vi "configuration UI.vi"() -> ()   [LabVIEW 2013, in "Tag Bus Web Interface editor node.lvclass"]
uses:
  Tag Bus Web Interface editor node.lvclass
  <vilib>/CEF_TreeControl/Node/NodeRef.ctl
  <vilib>/CEF_TreeControl/Node/NISE_CEF_Node.lvclass
  <vilib>/NI/AMC/Message Queue.ctl
  <vilib>/NI/AMC/Message.ctl
  <vilib>/NI/Tools/Keyed Array/KeyedArray.ctl
  <vilib>/CEF_TreeControl/Node/UserEventRef.ctl
  <vilib>/CEF_TreeControl/Controls/EventCluster.ctl
  <vilib>/NI/Module Execution Interface/Engine Configuration/engine configuration.lvclass
  <vilib>/NI/Tag Bus Data Framework/Configuration Editor/Classes/Engine Parent/Engine Parent Editor Node.lvclass
  <vilib>/NI/TBM Modules/TBWI/configuration/Tag Bus Web Interface configuration.lvclass
  <vilib>/NI/Tag Bus/tag/tag descriptor.lvclass
  <vilib>/NI/Tag Bus/tag/Data Type.ctl
  <vilib>/NI/Tag Bus/tag/tag descriptor.lvclass/tag descriptor.ctl
  Tag Bus Web Interface editor node.lvclass/Tag Bus Web Interface editor node.ctl
  <vilib>/NI/Tag Bus Module Framework/root configuration/TBM configuration.lvclass/TBM configuration.ctl
  <vilib>/NI/Tag Bus Module Framework/channel/channel classification.ctl
  <vilib>/NI/Tag Bus/tag/write tag name.vi
  <vilib>/NI/Tag Bus/tag/write data type.vi
  <vilib>/NI/Tag Bus/tag/read tag name.vi
  <vilib>/NI/Tag Bus Data Framework/Configuration Editor/Classes/Engine Parent/read engine configuration.vi
  <vilib>/NI/Tag Bus Module Framework/root configuration/create GUID.vi
  <vilib>/NI/Tag Bus Data Framework/Configuration Editor/Classes/Engine Parent/write engine configuration.vi
  <vilib>/NI/Tag Bus Module Framework/root configuration/TBM configuration.lvclass
  <vilib>/NI/Tag Bus Data Framework/Configuration Editor/Classes/Module editor node/module editor node.lvclass
  <vilib>/CEF_TreeControl/NISE_CEF_TreeControl.lvlib
  <vilib>/NI/Tag Bus Module Framework/channel/TBM channel.lvclass
  <vilib>/NI/Tools/Keyed Array/Tools_KeyedArray.lvlib
  <vilib>/NI/AMC/AMC.lvlib
panel:
  in  "Tab Control":enum32{"Web Configuration"}(tab)
  in  "remove to":bool
  in  "add to":bool
  in  "remove from":bool
  in  "add from":bool
  in  "toTBWlist":i32(listbox)
  in  "fromTBWlist":i32(listbox)
  in  "avail tags":i32(listbox)=-1
  in  "Direction":enum32{"From TBWI", "To TBWI"}(radio)
  in  "user event":T1
  in  "main queue":T2
  in  "node ref":T3
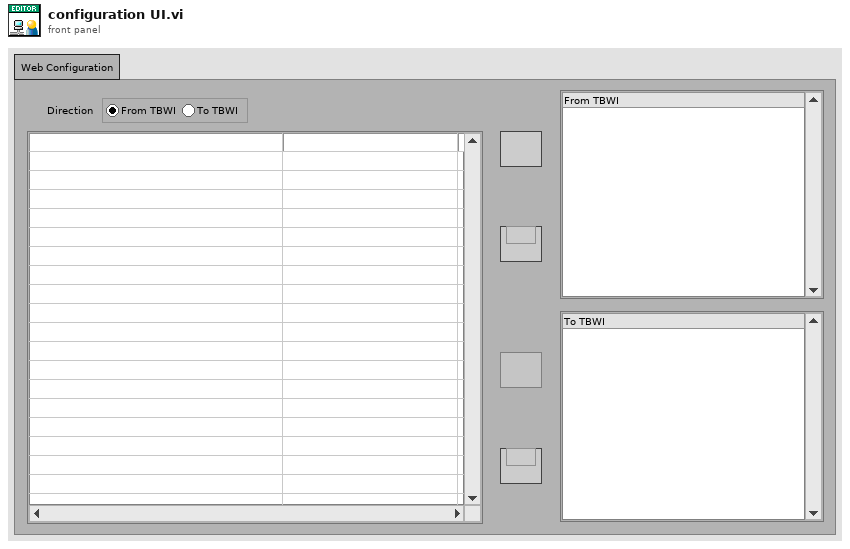
[diagram p1: front panel]
types:
  T1 = typedef "NISE_CEF_Node.lvclass/UserEventRef.ctl" = refnum<user-event>
  T2 = typedef "AMC.lvlib/Message Queue.ctl" = refnum<queue>
  T3 = typedef "NISE_CEF_Node.lvclass/NodeRef.ctl" = refnum<data-value>
  T4 = typedef "NISE_CEF_TreeControl.lvlib/EventCluster.ctl" = cluster{"command":string, "data":string}
  T5 = typedef "tag bus.lvlib/tag descriptor.lvclass/Data Type.ctl" = enum16{"Double", "Single", "I64", "I32", "I16", "I8", "U64", "U32", "U16", "U8", "Boolean", "String", "Array of Double", "Array of Single", "Array of I64", "Array of I32", "Array of I16", "Array of I8", "Array of U64", "Array of U32", "Array of U16", "Array of U8", "Array of Boolean", "Array of String"}
  T6 = enum8{"Enabled", "Disabled", "Disabled and Grayed Out"}
  T7 = typedef "TBM channel.lvclass/channel classification.ctl" = enum16{"input data", "output data", "processing parameter", "processing result"}
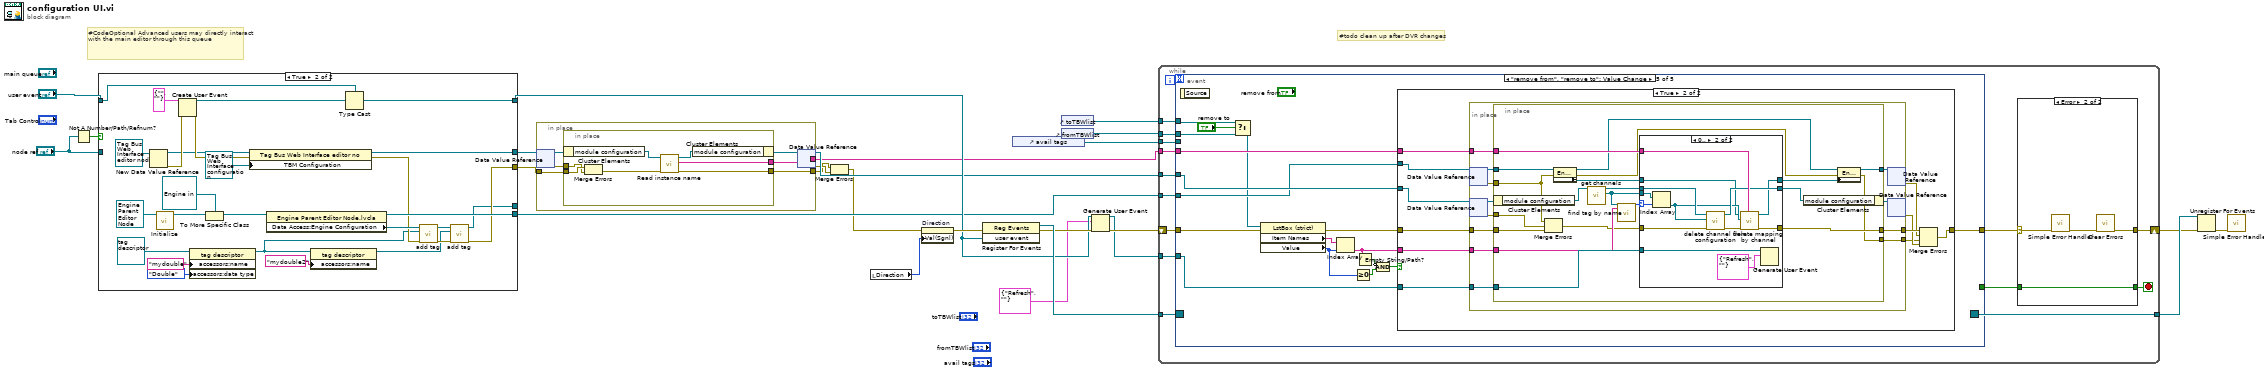
[diagram p0: block diagram]
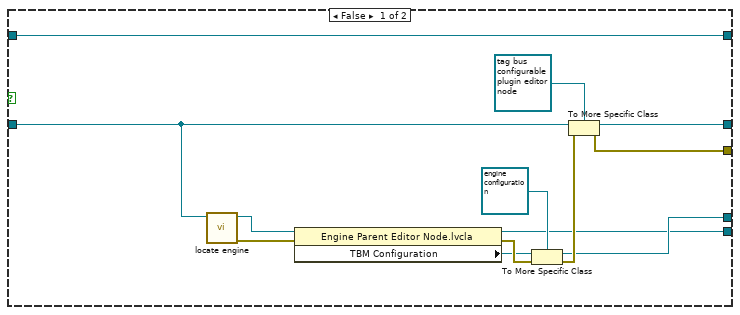
[diagram p2: hidden frame]
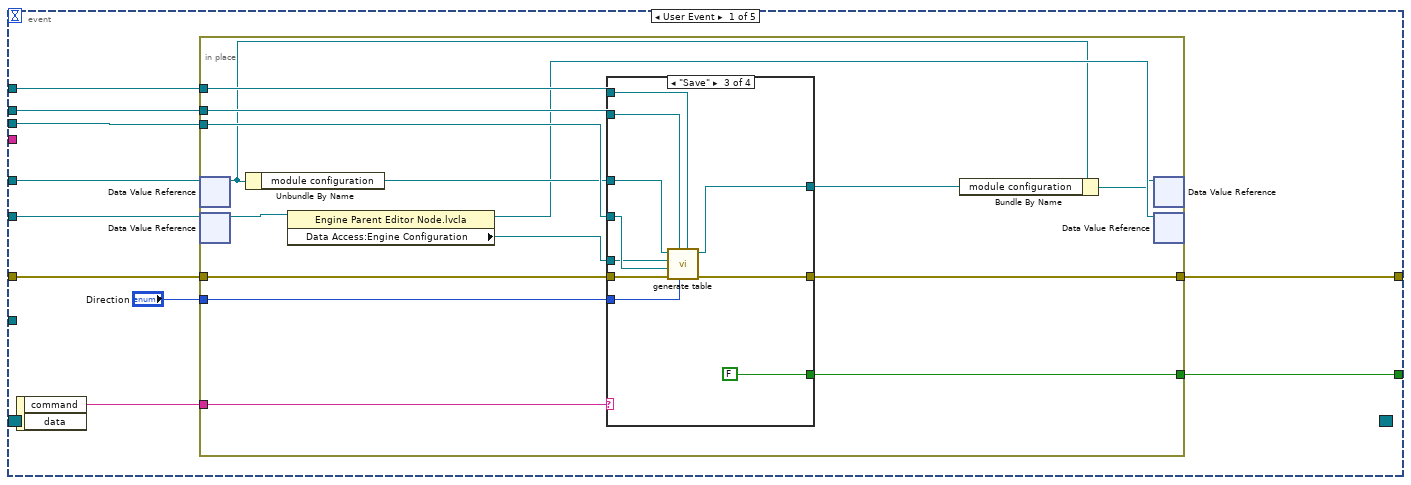
[diagram p4: hidden frame]
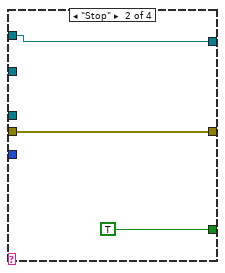
[diagram p6: hidden frame]
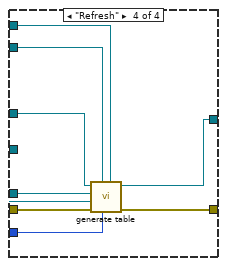
[diagram p7: hidden frame]
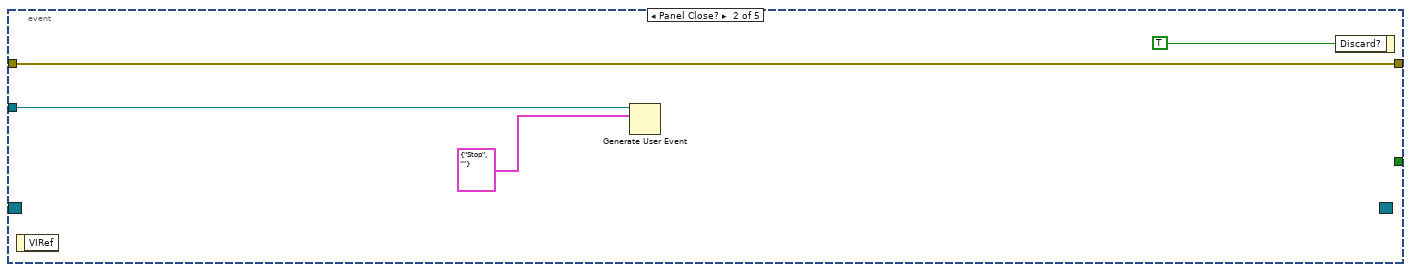
[diagram p8: hidden frame]
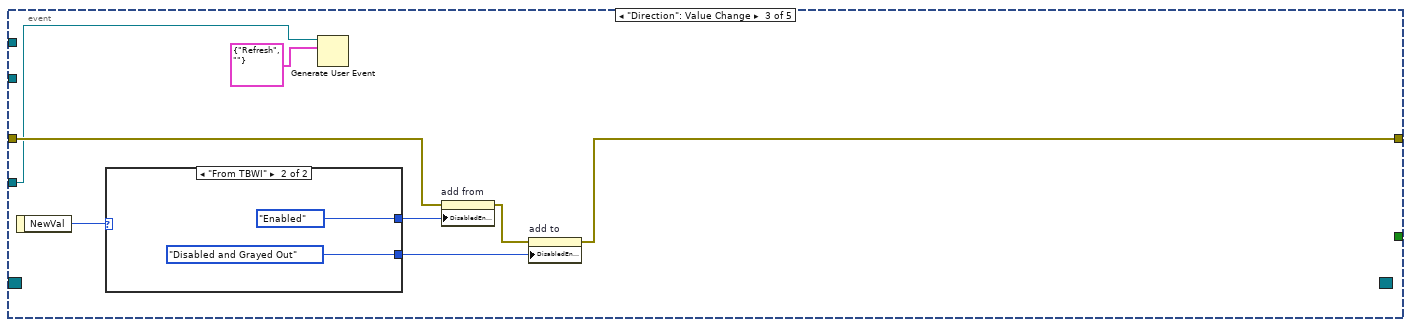
[diagram p9: hidden frame]
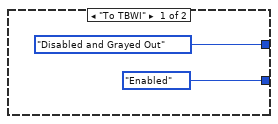
[diagram p10: hidden frame]
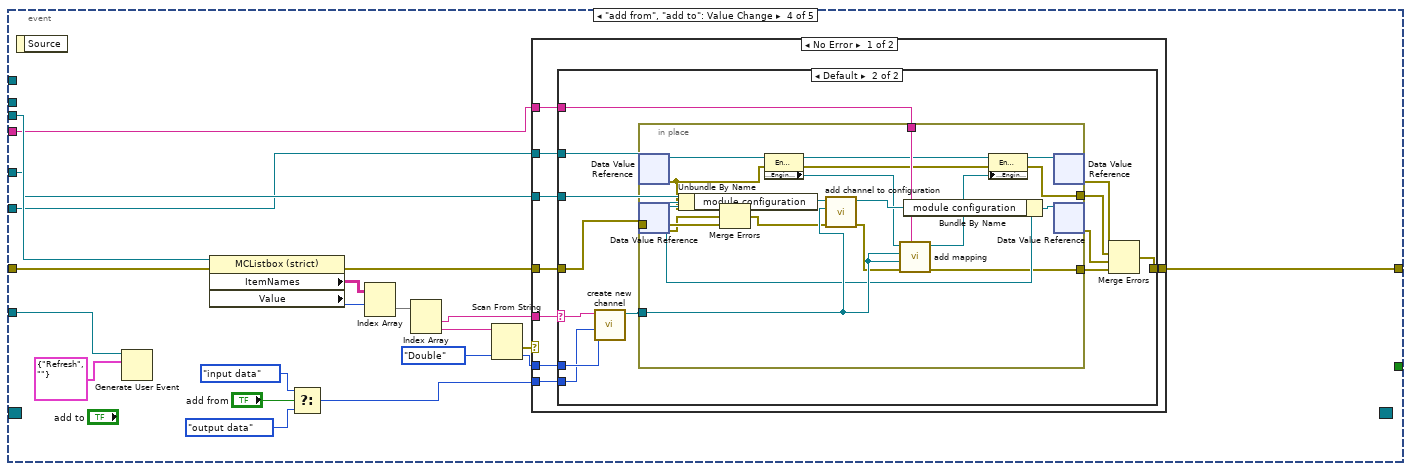
[diagram p11: hidden frame]
diagram:
  # "#todo clean up after DVR changes"
  # "#CodeOptional Advanced users may directly interact with the main editor through this queue"
  n1 = Not A Number/Path/Refnum?(number/path/refnum="node ref") -> (NaN/Path/Refnum?=w22:bool)
  n2 = case shown="True" w22 {
    tunnel: "user event" -> [w38 w39]
    tunnel: [w38 w40] -> w11
    tunnel: "node ref" -> [w36 _]
    tunnel: [w35 w59] -> w7
    tunnel: [w34 w44] -> w5
    tunnel: [w27 w43] -> _
    tunnel: [w26 w53] -> w8
    frame False {
      n3 = call <vilib>:"locate engine.vi"("component"=w36) -> ("error out"=w31:errorcluster, "engine"=w33:refnum<data-value>)  [unwired: 9 in]
      n4 = property class="Engine Parent Editor Node.lvcla"(reference=w33, error in=w31) -> (reference out=w26:refnum<data-value>, error out=w30:errorcluster, "TBM Configuration"=w29:refnum<class "TBM configuration.lvclass">)
      n5 = To More Specific Class(target class=refnum<class "engine configuration.lvclass"> refnum ("engine configuration.lvclass"), reference=w29, error in=w30) -> (specific class reference=w27:refnum<class "engine configuration.lvclass">, error out=w28:errorcluster)
      n6 = To More Specific Class(target class=refnum<data-value> refnum ("data value reference"), reference=w36, error in=w28) -> (specific class reference=w35:refnum<data-value>, error out=w34:errorcluster)
    }
    frame True {
      n7 = New Data Value Reference(data value=refnum<class "Tag Bus Web Interface editor node.lvclass"> refnum ("tag bus configurable plugin editor node")) -> (data value reference=w58:refnum<data-value>, error out=w61:errorcluster)  [unwired: 1 in]
      n8 = call-dynamic "Initialize.vi"("Engine in"=refnum<class "Engine Parent Editor Node.lvclass"> refnum) -> ("data value reference"=w57:T3)  [unwired: 8 in, 2 out]
      n9 = Create User Event(user event datatype=T4 {"command"="", "data"=""} ("event data"), error in=w61) -> (user event=w64:refnum<user-event>, error out=w60:errorcluster)
      n10 = property class="tag descriptor"(reference=refnum<class "tag descriptor.lvclass"> refnum ("tag descriptor"), "accessors:name"="mydouble" ("name"), "accessors:data type"=Data_Type."Double" ("data type")) -> (reference out=w41:refnum<class "tag descriptor.lvclass">)  [unwired: 1 in, 1 out]
      n11 = To More Specific Class(target class=refnum<data-value> refnum ("data value reference"), reference=w57) -> (specific class reference=w56:refnum<data-value>)  [unwired: 1 in, 1 out]
      n12 = property class="Tag Bus Web Interface editor no"(reference=w58, error in=w60, "TBM Configuration"=refnum<class "Tag Bus Web Interface configuration.lvclass"> refnum ("tag bus configurable plugin module configuration")) -> (reference out=w59:refnum<data-value>, error out=w48:errorcluster)
      n13 = property class="Engine Parent Editor Node.lvcla"(reference=w56) -> (reference out=w53:refnum<data-value>, "Data Access:Engine Configuration"=w52:refnum<class "engine configuration.lvclass">)  [unwired: 1 in, 1 out]
      n14 = property class="tag descriptor"(reference=w41, "accessors:name"="mydouble2" ("name")) -> (reference out=w42:refnum<class "tag descriptor.lvclass">)  [unwired: 1 in, 1 out]
      n15 = Type Cast(type=w39, x=w64) -> (*(type *) &x=w40:T1)
      n16 = call <vilib>:"add tag.vi"("error in"=w48, "tag descriptor"=w41, "engine configuration in"=w52) -> ("error out"=w46:errorcluster, "engine configuration out"=w45:refnum<class "engine configuration.lvclass">)  [unwired: 7 in]
      n17 = call <vilib>:"add tag.vi"("error in"=w46, "tag descriptor"=w42, "engine configuration in"=w45) -> ("error out"=w44:errorcluster, "engine configuration out"=w43:refnum<class "engine configuration.lvclass">)  [unwired: 7 in]
    }
  }
  n18 = in-place {
    in-place-border: w5 -> [w69]
    in-place-border: [w68] -> w3
    in-place-border: [w67] -> w2
    n19 = in-place-dvr #1(w7) -> (w71:refnum<class "Tag Bus Web Interface editor node.lvclass">, w70:errorcluster)
    n20 = in-place {
      in-place-border: w70 -> [w77]
      in-place-border: w69 -> [w78]
      in-place-border: [w73] -> w68
      in-place-border: [w72] -> w67
      n21 = in-place-cluster #2(w71) -> ("module configuration"=w76:refnum<class "Tag Bus Web Interface configuration.lvclass">)
      n22 = Merge Errors(w78, w77) -> (w74:errorcluster)
      n23 = call <vilib>:"Read instance name.vi"("error in"=w74, "configuration in"=w76) -> ("error out"=w73:errorcluster, "instance id"=w72:string, "configuration out"=w75:refnum<class "Tag Bus Web Interface configuration.lvclass">)  [unwired: 7 in]
      n24 = in-place-cluster #2("module configuration"=w75) -> (w66:refnum<class "Tag Bus Web Interface editor node.lvclass">)
    }
    n25 = in-place-dvr #1(w66) -> (w6:refnum<data-value>, w4:errorcluster)
  }
  n26 = Merge Errors(w3, w4) -> (w1:errorcluster)
  n27 = local read "Direction"() -> (w13:enum32{"From TBWI", "To TBWI"})
  n28 = property on="Direction" class="RadioBtnsControl (strict)"(error in=w1, "Val(Sgnl)"=w13) -> (error out=w14:errorcluster)  [unwired: 1 in, 1 out]
  n29 = register-events(error in=w14, w11) -> (reference out=w25:refnum<event-registration>, error out=w19:errorcluster)  [unwired: 1 in]
  n30 = control-ref of="avail tags"() -> (w17:refnum<vi>)
  n31 = control-ref of="toTBWlist"() -> (w16:refnum<vi>)
  n32 = control-ref of="fromTBWlist"() -> (w15:refnum<vi>)
  n33 = Generate User Event(user event=w11, event data cluster=T4 {"command"="Refresh", "data"=""} ("event data"), error in=w19) -> (user event out=w10:T1, error out=w12:errorcluster)  [unwired: 1 in]
  n34 = while {
    tunnel: w25 -> [w92]
    tunnel: [w91] -> w24
    shift-right: [w87] -> w23
    shift-left: w12 -> [w90]
    tunnel: w2 -> [w84]
    tunnel: w17 -> [w82]
    tunnel: w10 -> [w81]
    tunnel: w16 -> [w80]
    tunnel: w15 -> [w79]
    tunnel: w6 -> [w86]
    tunnel: w8 -> [w85]
    stop <- w89 stop-if-true
    n35 = event shown="[4] \"remove from\", \"remove to\": Value Change" {
      selector: w92 -> [_ _ _ _ _]
      dyn-events: [_ _ _ _ _] -> w91
      timeout: _ -> [_ _ _ _ _]
      tunnel: [w108 _ _ _ _] -> w88
      tunnel: [w106 w151 w154 w165 w233] -> w83
      tunnel: w90 -> [w105 w151 w155 w170 w228]
      tunnel: w86 -> [w100 _ _ w168 w232]
      tunnel: w85 -> [w99 _ _ w167 w231]
      tunnel: w84 -> [_ _ _ w166 w230]
      tunnel: w82 -> [w104 _ _ w169 _]
      tunnel: w81 -> [_ w149 w152 w184 w227]
      tunnel: w80 -> [w102 _ _ _ w243]
      tunnel: w79 -> [w103 _ _ _ w241]
      event User Event {
        n36 = event-data() -> ("command"=w107:string)  [unwired: 1 in, 1 out]
        n37 = in-place {
          in-place-border: [w123] -> w108
          in-place-border: w107 -> [w122]
          in-place-border: [w121] -> w106
          in-place-border: w105 -> [w120]
          in-place-border: w104 -> [w119]
          in-place-border: w103 -> [w118]
          in-place-border: w102 -> [w117]
          in-place-border: "Direction" -> [w116]
          n38 = in-place-dvr #3(w100) -> (w111:refnum<class "Tag Bus Web Interface editor node.lvclass">)  [unwired: 1 out]
          n39 = in-place-dvr #4(w99) -> (w115:refnum<class "Engine Parent Editor Node.lvclass">)  [unwired: 1 out]
          n40 = Unbundle By Name(w111) -> ("module configuration"=w114:refnum<class "Tag Bus Web Interface configuration.lvclass">)
          n41 = property class="Engine Parent Editor Node.lvcla"(reference=w115) -> (reference out=w112:refnum<class "Engine Parent Editor Node.lvclass">, "Data Access:Engine Configuration"=w113:refnum<class "engine configuration.lvclass">)  [unwired: 1 in, 1 out]
          n42 = case shown="\"Save\"" w122 {
            tunnel: [_ TRUE FALSE _] -> w123
            tunnel: [w125 w127 w132 w146] -> w121
            tunnel: w120 -> [w125 w127 w137 w147]
            tunnel: w119 -> [_ _ w134 w142]
            tunnel: w118 -> [_ _ w135 w145]
            tunnel: w117 -> [_ _ w136 w144]
            tunnel: w116 -> [_ _ w133 w143]
            tunnel: w114 -> [w124 w126 w131 w140]
            tunnel: w113 -> [_ _ w130 w139]
            tunnel: [w124 w126 w129 w141] -> w110
            frame Default {
            }
            frame "Stop" {
            }
            frame "Save" {
              n43 = call "generate table.vi"("to tbwi"=w136, "Direction"=w133, "from tbwi"=w135, "error in"=w137, "tags"=w134, "engine configuration in"=w130, "Tag Bus Web Interface configuration in"=w131) -> ("error out"=w132:errorcluster, "TBWI Cfg out"=w129:refnum<class "Tag Bus Web Interface configuration.lvclass">)  [unwired: 3 in]
            }
            frame "Refresh" {
              n44 = call "generate table.vi"("to tbwi"=w144, "Direction"=w143, "from tbwi"=w145, "error in"=w147, "tags"=w142, "engine configuration in"=w139, "Tag Bus Web Interface configuration in"=w140) -> ("error out"=w146:errorcluster, "TBWI Cfg out"=w141:refnum<class "Tag Bus Web Interface configuration.lvclass">)  [unwired: 3 in]
            }
          }
          n45 = Bundle By Name(cluster=w111, "module configuration"=w110) -> (w109:refnum<class "Tag Bus Web Interface editor node.lvclass">)
          n46 = in-place-dvr #3(w109) -> ()  [unwired: 2 out]
          n47 = in-place-dvr #4(w112) -> ()  [unwired: 2 out]
        }
      }
      event Panel Close? {
        n48 = event-data() -> ()  [unwired: 1 in, 1 out]
        n49 = Generate User Event(user event=w149, event data cluster=T4 {"command"="Stop", "data"=""} ("event data")) -> ()  [unwired: 2 in, 2 out]
        n50 = event-data("Discard?"=TRUE) -> ()  [unwired: 1 in, 1 out]
      }
      event "Direction": Value Change {
        n51 = event-data() -> ("NewVal"=w159:enum32{"From TBWI", "To TBWI"})  [unwired: 1 in]
        n52 = case shown="\"From TBWI\"" w159 {
          tunnel: [T6."Disabled and Grayed Out" ("Disabled") T6."Enabled" ("Disabled")] -> w158
          tunnel: [T6."Enabled" ("Disabled") T6."Disabled and Grayed Out" ("Disabled")] -> w157
          frame "To TBWI" {
          }
          frame "From TBWI" {
          }
        }
        n53 = Generate User Event(user event=w152, event data cluster=T4 {"command"="Refresh", "data"=""} ("event data")) -> ()  [unwired: 2 in, 2 out]
        n54 = property on="add from" class="Bool"(error in=w155, "DisabledEnum"=w158) -> (error out=w156:errorcluster)  [unwired: 1 in, 1 out]
        n55 = property on="add to" class="Bool"(error in=w156, "DisabledEnum"=w157) -> (error out=w154:errorcluster)  [unwired: 1 in, 1 out]
      }
      event "add from", "add to": Value Change {
        n56 = event-data() -> ()  [unwired: 1 in, 1 out]
        n57 = Generate User Event(user event=w184, event data cluster=T4 {"command"="Refresh", "data"=""} ("event data")) -> ()  [unwired: 2 in, 2 out]
        n58 = property class="MCListbox (strict)"(reference=w169, error in=w170) -> (error out=w171:errorcluster, "ItemNames"=w172:string[][], "Value"=w173:i32)  [unwired: 1 out]
        n59 = Select(t=channel_classification."input data" ("channel classification"), s="add from", f=channel_classification."output data" ("channel classification")) -> (s? t:f=w164:T7)
        n60 = Index Array(array=w172, index (row)=w173) -> (element=w176:string[])  [unwired: 1 in]
        n61 = Index Array(array=w176) -> (element #1=w177:string, element #2=w174:string)  [unwired: 2 in]
        n62 = Scan From String(input string=w174, default 1=Data_Type."Double" ("data type")) -> (error out=w178:errorcluster, output 1=w179:T5)  [unwired: 3 in, 2 out]
        n63 = case shown="No Error" w178 {
          tunnel: [w192 w226] -> w165
          tunnel: w166 -> [w191 _]
          tunnel: w168 -> [w190 _]
          tunnel: w167 -> [w189 _]
          tunnel: w171 -> [w188 w226]
          tunnel: w177 -> [w187 _]
          tunnel: w179 -> [w186 _]
          tunnel: w164 -> [w185 _]
          frame No Error {
            n64 = case shown="Default" w187 {
              selector: w187 -> [_ w204]
              tunnel: [w193 w198] -> w192
              tunnel: w188 -> [w193 w206]
              tunnel: w189 -> [_ w199]
              tunnel: w190 -> [_ w200]
              tunnel: w191 -> [_ w205]
              tunnel: w186 -> [_ w203]
              tunnel: w185 -> [_ w201]
              frame "" {
              }
              frame Default {
                n65 = call <vilib>:"create new channel.vi"("channel classification"=w201, "data type"=w203, "channel name"=w204) -> ("channel"=w202:refnum<class "TBM channel.lvclass">)  [unwired: 8 in]
                n66 = in-place {
                  in-place-border: w206 -> [w225]
                  in-place-border: w205 -> [w224]
                  in-place-border: w202 -> [w223]
                  in-place-border: [w211] -> w195
                  in-place-border: [w207] -> w194
                  n67 = in-place-dvr #5(w199) -> (w217:refnum<class "Engine Parent Editor Node.lvclass">, w208:errorcluster)
                  n68 = in-place-dvr #6(w200) -> (w220:refnum<class "Tag Bus Web Interface editor node.lvclass">, w212:errorcluster)
                  n69 = Unbundle By Name(w220) -> ("module configuration"=w221:refnum<class "Tag Bus Web Interface configuration.lvclass">)
                  n70 = Merge Errors(w208, w212, w225) -> (w210:errorcluster)
                  n71 = property class="Engine Parent Editor Node.lvcla"(reference=w217, error in=w208) -> (reference out=w216:refnum<class "Engine Parent Editor Node.lvclass">, error out=w209:errorcluster, "Data Access:Engine Configuration"=w214:refnum<class "engine configuration.lvclass">)
                  n72 = call <vilib>:"add channel to configuration.vi"("error in"=w210, "TBM channel in"=w223, "Tag Bus Web Interface configuration in"=w221) -> ("error out"=w222:errorcluster, "Tag Bus Web Interface configuration out"=w218:refnum<class "Tag Bus Web Interface configuration.lvclass">)  [unwired: 7 in]
                  n73 = call <vilib>:"add mapping.vi"("owner ID"=w224, "error in"=w222, "channel"=w223, "tag descriptor"=w223, "engine configuration"=w214) -> ("error out"=w211:errorcluster, "engine configuration out"=w215:refnum<class "engine configuration.lvclass">)  [unwired: 5 in]
                  n74 = Bundle By Name(cluster=w220, "module configuration"=w218) -> (w219:refnum<class "Tag Bus Web Interface editor node.lvclass">)
                  n75 = property class="Engine Parent Editor Node.lvcla"(reference=w216, error in=w209, "Data Access:Engine Configuration"=w215) -> (reference out=w213:refnum<class "Engine Parent Editor Node.lvclass">, error out=w207:errorcluster)
                  n76 = in-place-dvr #5(w213) -> (w197:errorcluster)  [unwired: 1 out]
                  n77 = in-place-dvr #6(w219) -> (w196:errorcluster)  [unwired: 1 out]
                }
                n78 = Merge Errors(w197, w194, w196, w195) -> (w198:errorcluster)
              }
            }
          }
          frame Error {
          }
        }
      }
      event "remove from", "remove to": Value Change {
        n79 = event-data() -> ()  [unwired: 1 in, 1 out]
        n80 = Select(t=w243, s="remove to", f=w241) -> (s? t:f=w229:refnum<vi>)
        n81 = property class="LstBox (strict)"(reference=w229, error in=w228) -> (error out=w239:errorcluster, "Item Names"=w234:string[], "Value"=w235:i32)  [unwired: 1 out]
        n82 = Index Array(array=w234, index=w235) -> (element=w240:string)
        n83 = Greater Or Equal To 0?(x=w235) -> (x >= 0?=w237:bool)
        n84 = Empty String/Path?(string/path=w240) -> (empty?=w236:bool)
        n85 = Compound Arithmetic op=AND(invert w236, w237) -> (w238:bool)
        n86 = case shown="True" w238 {
          tunnel: w239 -> [w244 w252]
          tunnel: [w244 w248] -> w233
          tunnel: w232 -> [_ w250]
          tunnel: w231 -> [_ w249]
          tunnel: w227 -> [_ w255]
          tunnel: w240 -> [_ w254]
          tunnel: w230 -> [_ w251]
          frame False {
          }
          frame True {
            n87 = in-place {
              in-place-border: w255 -> [w267]
              in-place-border: w254 -> [w266]
              in-place-border: [w265] -> w253
              in-place-border: w252 -> [w264]
              in-place-border: w251 -> [w263]
              in-place-border: [w256] -> w245
              n88 = in-place-dvr #7(w249) -> (w258:refnum<class "Engine Parent Editor Node.lvclass">, w260:errorcluster)
              n89 = in-place-dvr #8(w250) -> (w262:refnum<class "Tag Bus Web Interface editor node.lvclass">, w259:errorcluster)
              n90 = in-place {
                in-place-border: w267 -> [w287]
                in-place-border: w266 -> [w286]
                in-place-border: [w283] -> w265
                in-place-border: w264 -> [w282]
                in-place-border: w263 -> [w280]
                in-place-border: w260 -> [w268]
                in-place-border: w259 -> [w276]
                in-place-border: w258 -> [w275]
                in-place-border: [w274] -> w257
                in-place-border: [w270] -> w256
                n91 = in-place-cluster #9(w262) -> ("module configuration"=w278:refnum<class "Tag Bus Web Interface configuration.lvclass">)
                n92 = Merge Errors(w268, w276, w282) -> (w277:errorcluster)
                n93 = property class="Engine Parent Editor Node.lvcla"(reference=w275, error in=w268) -> (reference out=w273:refnum<class "Engine Parent Editor Node.lvclass">, error out=w269:errorcluster, "Data Access:Engine Configuration"=w272:refnum<class "engine configuration.lvclass">)
                n94 = call-dynamic "get channels.vi"("Tag Bus Web Interface configuration in"=w278) -> ("channels"=w281:refnum<class "TBM channel.lvclass">[], "Tag Bus Web Interface configuration out"=w284:refnum<class "Tag Bus Web Interface configuration.lvclass">)  [unwired: 9 in]
                n95 = call <vilib>:"find tag by name.vi"("name"=w286, "tags in"=w281) -> ("index"=w285:i32)  [unwired: 9 in]
                n96 = case shown="0.." w285 {
                  selector: w285 -> [_ w301]
                  tunnel: w287 -> [_ w302]
                  tunnel: w284 -> [w290 w299]
                  tunnel: [w290 w295] -> w279
                  tunnel: [w289 w294] -> w283
                  tunnel: w277 -> [w289 w298]
                  tunnel: w281 -> [_ w300]
                  tunnel: w280 -> [_ w296]
                  tunnel: w272 -> [w288 w292]
                  tunnel: [w288 w291] -> w271
                  frame ..-1 {
                  }
                  frame 0.. {
                    n97 = Index Array(array=w300, index=w301) -> (element=w293:refnum<class "TBM channel.lvclass">)
                    n98 = call <vilib>:"delete channel from configuration.vi"("error in"=w298, "TBM channel in"=w293, "Tag Bus Web Interface configuration in"=w299) -> ("error out"=w297:errorcluster, "Tag Bus Web Interface configuration out"=w295:refnum<class "Tag Bus Web Interface configuration.lvclass">)  [unwired: 7 in]
                    n99 = call <vilib>:"delete mapping by channel.vi"("owner ID"=w296, "error in"=w297, "channel"=w293, "engine configuration in"=w292) -> ("error out"=w294:errorcluster, "engine configuration out"=w291:refnum<class "engine configuration.lvclass">)  [unwired: 6 in]
                    n100 = Generate User Event(user event=w302, event data cluster=T4 {"command"="Refresh", "data"=""} ("event data")) -> ()  [unwired: 2 in, 2 out]
                  }
                }
                n101 = in-place-cluster #9("module configuration"=w279) -> (w261:refnum<class "Tag Bus Web Interface editor node.lvclass">)
                n102 = property class="Engine Parent Editor Node.lvcla"(reference=w273, error in=w269, "Data Access:Engine Configuration"=w271) -> (reference out=w274:refnum<class "Engine Parent Editor Node.lvclass">, error out=w270:errorcluster)
              }
              n103 = in-place-dvr #7(w257) -> (w247:errorcluster)  [unwired: 1 out]
              n104 = in-place-dvr #8(w261) -> (w246:errorcluster)  [unwired: 1 out]
            }
            n105 = Merge Errors(w253, w247, w245, w246) -> (w248:errorcluster)
          }
        }
      }
    }
    n106 = case shown="Error" w83 {
      selector: w83 -> [w93 w97]
      tunnel: [w94 w98] -> w89
      tunnel: w88 -> [w94 w98]
      tunnel: [w93 w95] -> w87
      frame No Error {
      }
      frame Error {
        n107 = call <vilib>:"Simple Error Handler.vi"("error in (no error)"=w97) -> ("error out"=w96:errorcluster)  [unwired: 4 in, 4 out]
        n108 = call <vilib>:"Clear Errors.vi"("error in (no error)"=w96) -> ("error out"=w95:errorcluster)  [unwired: 6 in]
      }
    }
  }
  n109 = Unregister For Events(event registration refnum=w24, error in=w23) -> (error out=w18:errorcluster)
  n110 = call <vilib>:"Simple Error Handler.vi"("error in (no error)"=w18) -> ()  [unwired: 4 in, 5 out]
